vi "from string.vi"(8 "error in":errorcluster, 9 "data":string, 10 "version":string, 11 "module configuration in":refnum<class "TBM module configuration.lvclass">) -> (0 "error out":errorcluster, 3 "module configuration out":refnum<class "TBM module configuration.lvclass">)   [LabVIEW 2014, in "TBM module configuration.lvclass"]
doc: "Provides an interface for loading a module configuration from a file or other serialized data source. It is recommended that all children of this class store data in two sets--data required for its own initialization, and any data required for parent initialization--and that each implementation uses the <b>Call Parent Method</b> primitive to de-serialize parent information. As a result, it is expected that every module configuration class calls <b>component configuration.lvclass:From String.vi</b>."
uses:
  TBM module configuration.lvclass
  root configuration/TBM configuration.lvclass
  <vilib>/NI/Configuration Framework/serializable configuration/NISE_CEF_serializable configuration.lvclass
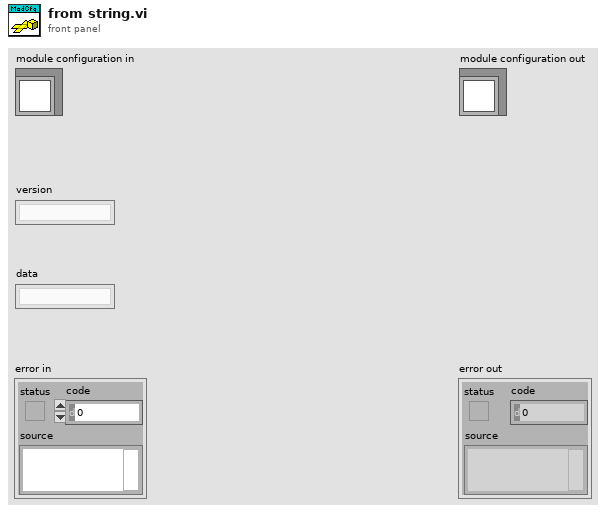
[diagram p1: front panel]
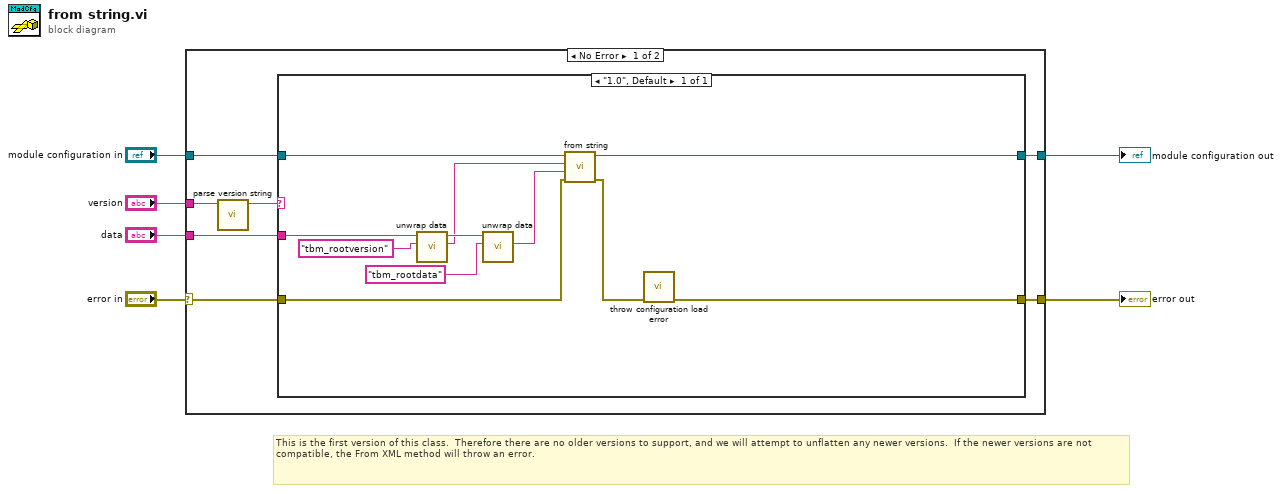
[diagram p0: block diagram]
diagram:
  # "This is the first version of this class.  Therefore there are no older versions to support, and we will attempt to unflatten any newer versions.  If the newer versions are not compatible, the From XML method will throw an error."
  n1 = case shown="No Error" "error in" {
    selector: "error in" -> [w7 w26]
    tunnel: "data" -> [w13 _]
    tunnel: "module configuration in" -> [w12 w25]
    tunnel: [w11 w25] -> w4
    tunnel: [w10 w26] -> w3
    tunnel: "version" -> [w9 _]
    frame No Error {
      n2 = call <vilib>:"parse version string.vi"("full version"=w9) -> ("major.minor version"=w8:string)  [unwired: 7 in, 3 out]
      n3 = case shown="\"1.0\", Default" w8 {
        tunnel: w13 -> [w23]
        tunnel: w7 -> [w14]
        tunnel: w12 -> [w24]
        tunnel: [w22] -> w11
        tunnel: [w15] -> w10
        frame "1.0", Default {
          n4 = call <vilib>:"unwrap data.vi"("identifier"="tbm_rootversion" ("additional identifier"), "data to unwrap"=w23) -> ("unwrapped data"=w17:string, "remaining string"=w19:string)  [unwired: 8 in]
          n5 = call <vilib>:"unwrap data.vi"("identifier"="tbm_rootdata" ("additional identifier"), "data to unwrap"=w19) -> ("unwrapped data"=w18:string)  [unwired: 8 in, 1 out]
          n6 = call-parent "from string.vi"("error in"=w14, "data"=w18, "version"=w17, "configuration in"=w24) -> ("error out"=w16:errorcluster, "configuration out"=w22:refnum<class "TBM module configuration.lvclass">)  [unwired: 6 in]
          n7 = call "throw configuration load error.vi"("error in"=w16) -> ("error out"=w15:errorcluster)  [unwired: 10 in]
        }
      }
    }
    frame Error {
    }
  }
  "error out" <- w3
  "module configuration out" <- w4
